vi "Termperature DAQ.vi"() -> ()   [LabVIEW 2011]
uses:
  <vilib>/Platform/TimedLoop/XDataNode/timing_clust.ctl
  <vilib>/Platform/TimedLoop/XDataNode/nitl_modes.ctl
  <vilib>/Platform/TimedLoop/XDataNode/wakeup.ctl
  <vilib>/DAQmx/read.llb/DAQmx Read (Analog DBL 1Chan 1Samp).vi
  <vilib>/DAQmx/create/channels.llb/DAQmx Create Channel (AI-Voltage-Basic).vi
  <vilib>/DAQmx/miscellaneous.llb/DAQmx Fill In Error Info.vi
  <vilib>/Platform/TimedLoop/XDataNode/XDataNode.xnode
  <vilib>/Platform/TimedLoop/XDataNode/XDNodeRunTimeDep.lvlib
panel:
  out "temp":dbl(slide) scale=-100.0..500.0
  in  "Fareight":bool
  out "iteration index":i32
  in  "?":bool
  out "DAQ Error":errorcluster
  out "Voltage":dbl format="%0.2f"
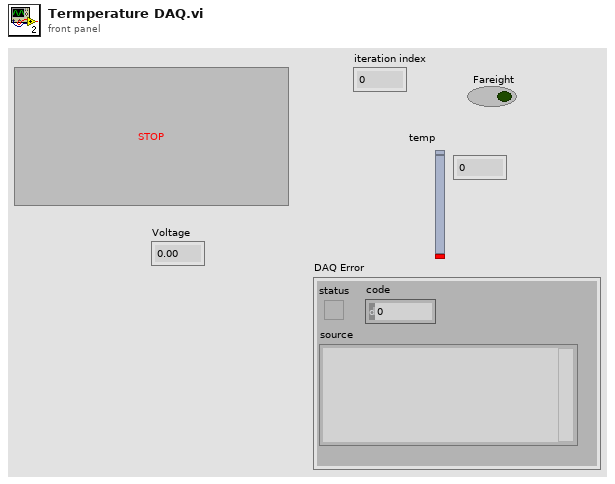
[diagram p1: front panel]
types:
  T1 = typedef "XDNodeRunTimeDep.lvlib/timing_clust.ctl" = cluster{"Expected End [f-1]":u64, "Actual End [f-1]":u64, "Finished Late? [f-1]":bool, "Expected End [i-1]":u64, "Actual End [i-1]":u64, "Finished Late? [i-1]":bool, "Expected Start [i]":u64, "Actual Start [i]":u64, "Expected Start [f]":u64, "Actual Start [f]":u64, "Source Name":string, "Structure Name":string, "Period":i64, "Deadline":i64, "Offset":i64, "Start":i64, "Priority":i32, "Timeout":i32, "Mode":T2, "Wakeup Reason":T3, "Error":errorcluster, "Source Type":string, "Secondary Source Type":string, "Global End Time":u64, "Global Start Time":u64, "Frame Duration":u64, "Iteration Duration":u64, "Assigned CPU":i32, "I/O Scan Engine Mode":u32}
  T2 = typedef "XDNodeRunTimeDep.lvlib/nitl_modes.ctl" = enum32{"No Change", "Process missed periods, maintain original phase", "Discard missed periods, maintain original phase", "Process missed periods, ignore original phase", "Discard missed periods, ignore original phase"}
  T3 = typedef "XDNodeRunTimeDep.lvlib/wakeup.ctl" = enum32{"Normal", "Aborted", "Asynchronous wakeup", "Timing source error", "Timed loop error", "Timeout"}
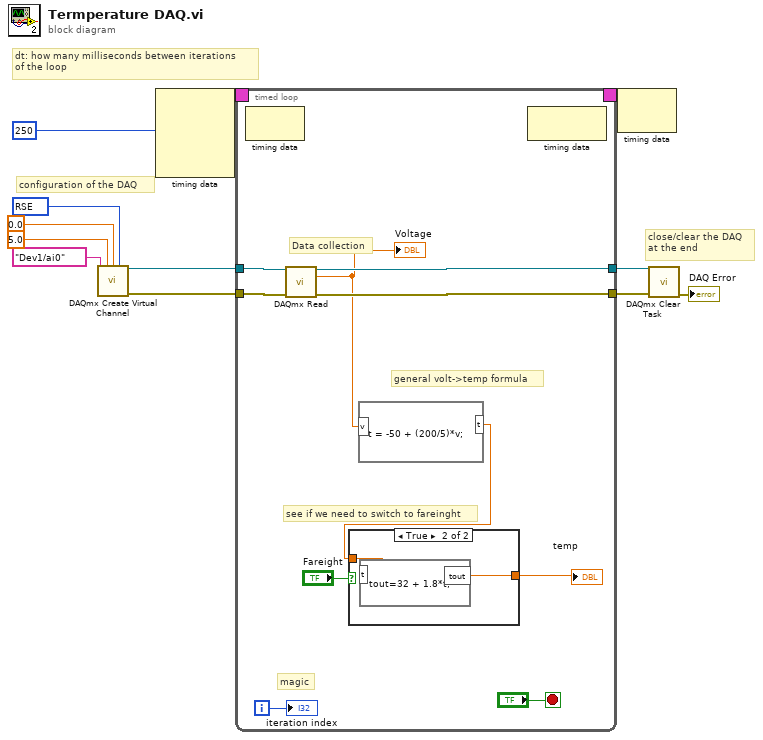
[diagram p0: block diagram]
diagram:
  w5 = 10083 items=["default"=-1, "RSE"=10083, "NRSE"=10078, "Differential"=10106, "Pseudodifferential"=12529] ("input terminal configuration")
  # "close/clear the DAQ\nat the end"
  # "configuration of the DAQ"
  # "dt: how many milliseconds between iterations\nof the loop"
  n1 = call-poly <vilib>:"DAQmx Create Virtual Channel.vi"("maximum value"=5.0, "minimum value"=0.0, "input terminal configuration"=w5, "physical channels"=tag "Dev1/ai0") -> ("task out"=w12:refnum<k21>, "error out"=w10:errorcluster)  [unwired: 10 in]
  n2 = node-c288(i64 250 ("Period")) -> (w3:T1)  [unwired: 3 in]
  n3 = timed-loop {
    timing: w3 -> [_]
    timing-out: [_] -> w2
    tunnel: w12 -> [w22]
    tunnel: [w21] -> w11
    tunnel: w10 -> [w20]
    tunnel: [w19] -> w9
    i -> [w17]
    stop <- "?" stop-if-true
    # "magic"
    # "see if we need to switch to fareinght"
    # "general volt->temp formula"
    # "Data collection"
    n4 = node-c288() -> ()  [unwired: 1 in, 1 out]
    n5 = call-poly <vilib>:"DAQmx Read.vi"("task/channels in"=w22, "error in"=w20) -> ("task out"=w21:refnum<k21>, "data"=w16:dbl, "error out"=w19:errorcluster)  [unwired: 11 in]
    "Voltage" <- w16
    n6 = formula code="t = -50 + (200/5)*v;"("v"=w16) -> ("t"=w14:dbl)
    n7 = case shown="True" "Fareight" {
      tunnel: w14 -> [w23 w25]
      tunnel: [w23 w24] -> w13
      frame False {
      }
      frame True {
        n8 = formula code="tout=32 + 1.8*t;"("t"=w25) -> ("tout"=w24:dbl)
      }
    }
    "temp" <- w13
    n9 = node-c288() -> ()  [unwired: 1 in, 1 out]
    "iteration index" <- w17
  }
  n10 = node-c288(w2) -> ()  [unwired: 1 out]
  n11 = call <vilib>:"DAQmx Clear Task.vi"("task in"=w11, "error in"=w9) -> ("error out"=→"DAQ Error":errorcluster)  [unwired: 13 in]
